vi "Test Read Servicio Estatus.vi"(8 "error in (no error)":errorcluster, 11 "TestCase in":refnum<class "Unit Testing.lvclass">) -> (0 "error out":errorcluster, 3 "TestCase out":refnum<class "Unit Testing.lvclass">)   [LabVIEW 2020, in "Unit Testing.lvclass"]
uses:
  Unit Testing.lvclass
  <vilib>/addons/_JKI Toolkits/VI Tester/TestCase.llb/TestCase.lvclass
  Contabilidad/Contabilidad.lvlib
  Manejador Turnos/Manejador Turnos.lvlib
  C:/Program Files (x86)/National Instruments/LabVIEW 2020/vi.lib/addons/_JKI Toolkits/VI Tester/TestCase.llb/TestCase.lvclass
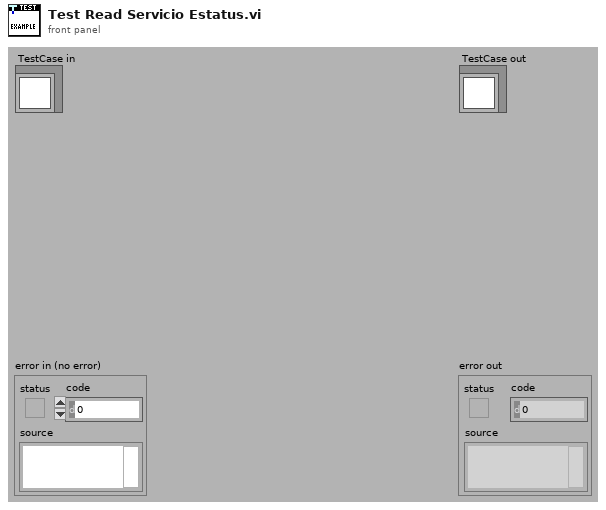
[diagram p1: front panel]
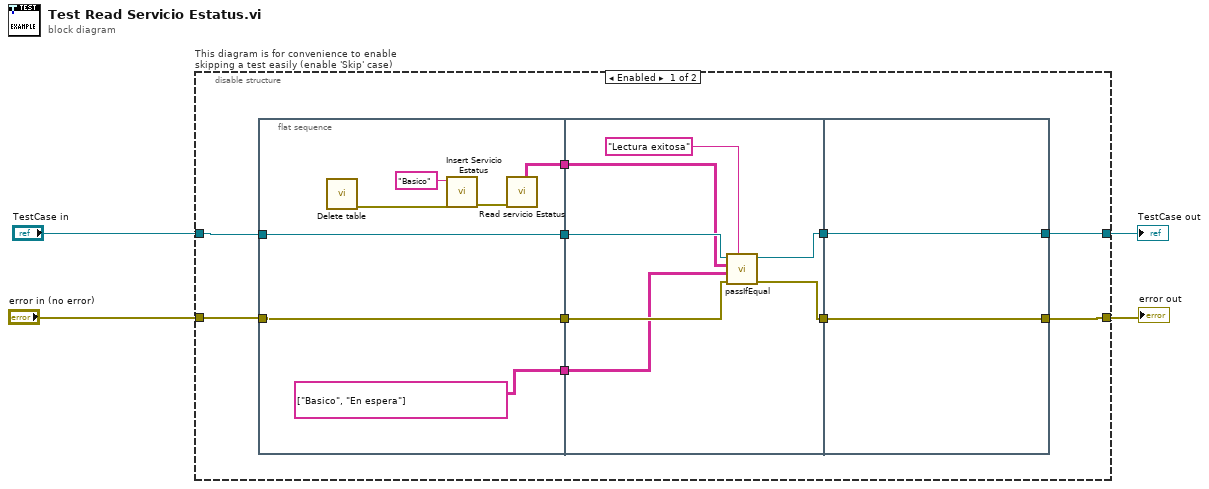
[diagram p0: block diagram]
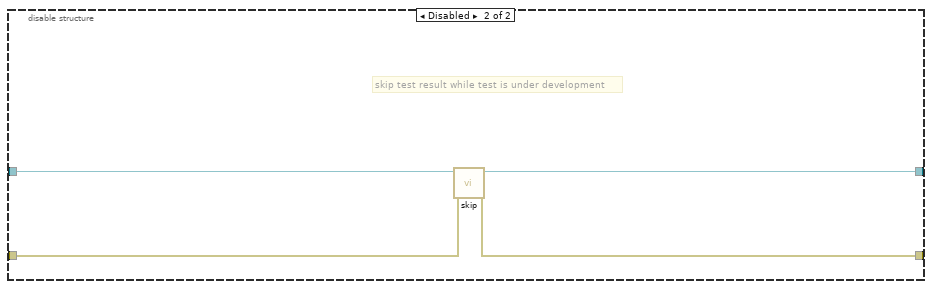
[diagram p2: hidden frame]
diagram:
  n1 = disable-structure "This diagram is for convenience to enable skipping a test easily (enable 'Skip' case)" shown="Enabled" {
    disable-tunnel: "TestCase in" -> [w8 w34]
    disable-tunnel: [w5 w32] -> w1
    disable-tunnel: [w6 w33] -> w3
    disable-tunnel: "error in (no error)" -> [w7 w31]
    frame Enabled {
      n2 = flat-sequence {
        tunnel: [w21] -> w14
        tunnel: w8 -> [w21]
        tunnel: [w20] -> w13
        tunnel: w7 -> [w20]
        tunnel: [w17] -> w12
        tunnel: [string[][] [["Basico", "En espera"]] ("Servicio Estatus")] -> w11
        tunnel: [w28] -> w10
        tunnel: [w27] -> w9
        tunnel: w14 -> [w26]
        tunnel: w13 -> [w25]
        tunnel: w12 -> [w24]
        tunnel: w11 -> [w23]
        tunnel: [w30] -> w5
        tunnel: w10 -> [w30]
        tunnel: [w29] -> w6
        tunnel: w9 -> [w29]
        frame #0 {
          n3 = call "Delete table.vi"() -> ("error out"=w16:errorcluster)  [unwired: 10 in, 1 out]
          n4 = call "Insert Servicio Estatus.vi"("error in (no error)"=w16, "Servicio"="Basico") -> ("error out"=w19:errorcluster)  [unwired: 9 in]
          n5 = call "Read servicio Estatus.vi"("error in (no error)"=w19) -> ("Servicio Estatus"=w17:string[][])  [unwired: 9 in, 1 out]
        }
        frame #1 {
          n6 = call-dynamic "passIfEqual.vi"("custom report message (\"\")"="Lectura exitosa" ("custom report message (\"\")"), "error in (no error)"=w25, "y"=w23, "x"=w24, "TestCase in"=w26) -> ("error out"=w27:errorcluster, "TestCase out"=w28:refnum<class "Unit Testing.lvclass">)  [unwired: 5 in]
        }
        frame #2 {
        }
      }
    }
    frame Disabled {
      # "skip test result while test is under development"
      n7 = call <vilib>:"skip.vi"("error in (no error)"=w31, "TestCase in"=w34) -> ("error out"=w33:errorcluster, "TestCase out"=w32:refnum<class "Unit Testing.lvclass">)  [unwired: 8 in]
    }
  }
  "error out" <- w3
  "TestCase out" <- w1
